vi "Измерения на 1 минуту.vi"() -> ()   [LabVIEW 2017]
panel:
  out "ladt temp":dbl
  out "Numeric":i32
  out "измеренная температура":dbl
  in  "ожидание (мс)":i32=500
  in  "количество итарераций":i32
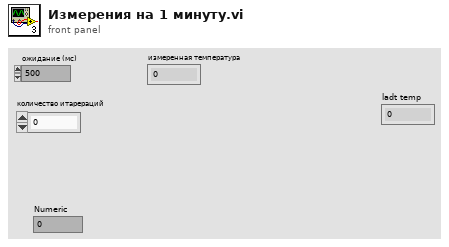
[diagram p1: front panel]
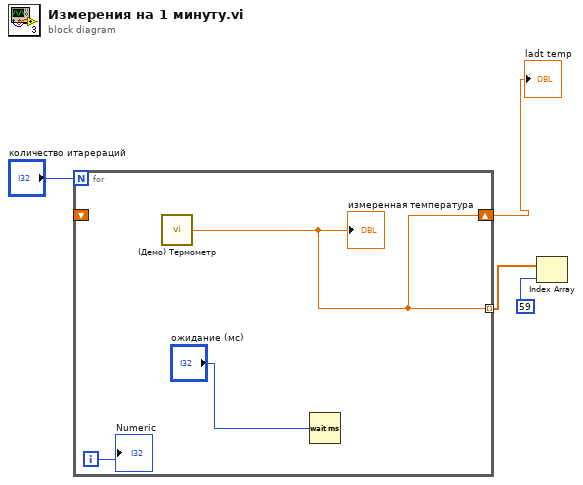
[diagram p0: block diagram]
diagram:
  n1 = for {
    N: "количество итарераций" -> [_]
    tunnel: [w5] -> w3 mode=indexing
    shift-right: [w5] -> w1
    shift-left: _ -> [_]
    i -> [w7]
    n2 = call "(Демо) Термометр.vi"() -> ("Температура"=w5:dbl)  [unwired: 1 in]
    "измеренная температура" <- w5
    n3 = Wait (ms)(milliseconds to wait="ожидание (мс)") -> ()  [unwired: 1 out]
    "Numeric" <- w7
  }
  "ladt temp" <- w1
  n4 = Index Array(array=w3, index=59) -> ()  [unwired: 1 out]
